vi "niRFUtil MT UTIL Perform Resampling (Complex SGL).vi"(0 "samples in":csg[](array[numeric]), 1 "effective filter length":i32, 2 "interpolation factor":i32, 3 "filterData":sgl[](array[numeric]), 5 "resampler state in":T1, 7 "offset":dbl, 9 "rate factor":dbl, 11 "error in (no error)":errorcluster, 12 "reset":bool=TRUE, 13 "flush":bool) -> (4 "samples out":csg[](array[numeric]), 6 "resampler state in":T1 caption="resampler state out", 15 "error out":errorcluster)   [LabVIEW 2015, in "niRFUtil.lvlib"]
uses:
  niRFUtil.lvlib
  Includes/niRFUtil MT INC Resampler State (Complex SGL).ctl
  niRFAMT.dll
panel:
  out "return value":i32
  # "This is Ts'/Ts"
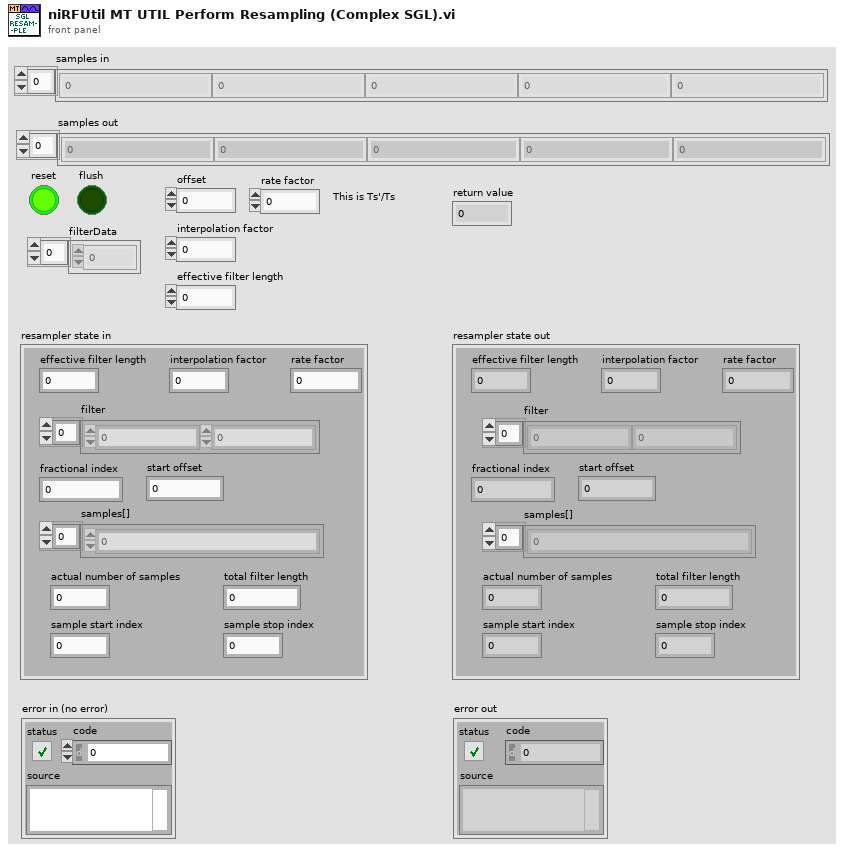
[diagram p1: front panel]
types:
  T1 = typedef "niRFUtil.lvlib/niRFUtil MT INC Resampler State (Complex SGL).ctl" = cluster{"effective filter length":i32, "interpolation factor":i32, "rate factor":dbl, "filter":sgl[], "fractional index":dbl, "start offset":i32, "samples[]":csg[], "actual number of samples":i32, "total filter length":i32, "sample start index":i32, "sample stop index":i32}
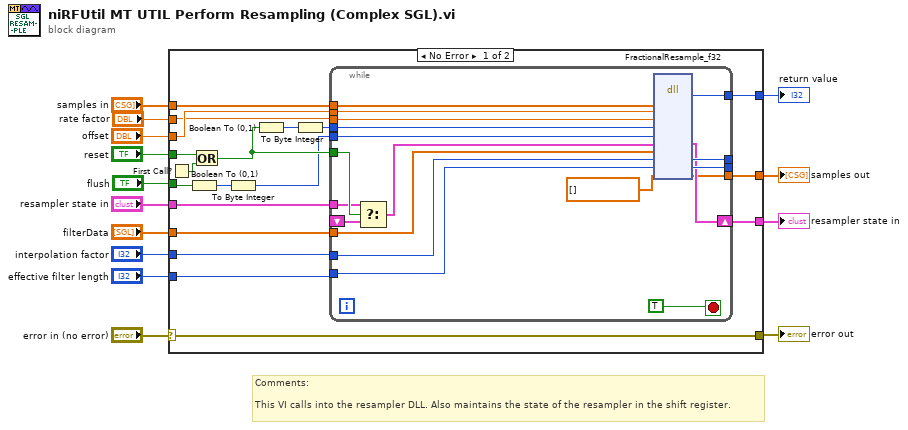
[diagram p0: block diagram]
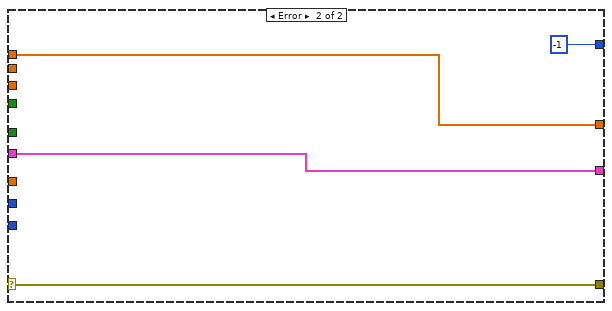
[diagram p2: hidden frame]
diagram:
  # "Comments:\n\nThis VI calls into the resampler DLL. Also maintains the state of the resampler in the shift register."
  n1 = case shown="No Error" "error in (no error)" {
    selector: "error in (no error)" -> [w24 w53]
    tunnel: "samples in" -> [w23 w56]
    tunnel: "resampler state in" -> [w20 w55]
    tunnel: [w33 w55] -> w12
    tunnel: "offset" -> [w32 _]
    tunnel: "reset" -> [w31 _]
    tunnel: "filterData" -> [w28 _]
    tunnel: "interpolation factor" -> [w27 _]
    tunnel: "effective filter length" -> [w26 _]
    tunnel: [w15 w56] -> w6
    tunnel: [w25 -1 ("return type")] -> w5
    tunnel: [w24 w53] -> w3
    tunnel: "rate factor" -> [w19 _]
    tunnel: "flush" -> [w17 _]
    frame No Error {
      n2 = First Call?() -> (First Call?: T/F=w22:bool)
      n3 = Boolean To (0,1)(Boolean=w17) -> (0, 1=w18:i16)
      n4 = Or(x=w31, y=w22) -> (x .or. y?=w21:bool)
      n5 = To Byte Integer(number=w18) -> (8bit integer=w16:i8)
      n6 = Boolean To (0,1)(Boolean=w21) -> (0, 1=w30:i16)
      n7 = To Byte Integer(number=w30) -> (8bit integer=w29:i8)
      n8 = while {
        tunnel: w32 -> [w52]
        tunnel: w29 -> [w44]
        tunnel: w28 -> [w39]
        tunnel: w27 -> [w40]
        tunnel: w26 -> [w41]
        tunnel: [w51] -> _
        tunnel: [w50] -> w25
        tunnel: w23 -> [w49]
        shift-right: [w37] -> w33
        shift-left: _ -> [w46]
        tunnel: w21 -> [w47]
        tunnel: w20 -> [w45]
        tunnel: w19 -> [w43]
        tunnel: [w42] -> _
        tunnel: w16 -> [w36]
        tunnel: [w35] -> w15
        stop <- TRUE stop-if-true
        n9 = Select(t=w45, s=w47, f=w46) -> (s? t:f=w38:T1)
        n10 = dll-call lib="C:/Perforce/semoore-sales/Customers/NATI-3813/Noise Floor/LV Filters/ParallelComplexFilterRFUtil/niRFUtil/MT/Utilities/niRFAMT.*" fn="FractionalResample_f32" ("FractionalResampler.dll:FractionalResampleWithNoRateChange")("samples in"=w49, "offset"=w52, "rateFactor"=w43, "reset"=w44, "flush"=w36, "state"=w38, "filterData"=w39, "interpolation factor"=w40, "effective filter length"=w41, csg[] [] ("samples in")) -> ("return type"=w50:i32, "state"=w37:T1, "interpolation factor"=w51:i32, "effective filter length"=w42:i32, w35:csg[])  [unwired: 9 in, 2 out]
      }
    }
    frame Error {
    }
  }
  "samples out" <- w6
  "resampler state in" <- w12
  "return value" <- w5
  "error out" <- w3
